vi "DP-Init Level Series.vi"(0 "state":T2, 1 "DP Freqs":T6, 5 "Parameters":T3, 11 "error in (no error)":errorcluster) -> (8 "level series":T1, 14 "Nominal f2 SPL":dbl[](array[numeric]), 15 "error out":errorcluster)   [LabVIEW 2020]
uses:
  Typedefs/DP-Freqs.ctl
  Typedefs/DP-Parameters.ctl
  Typedefs/DP-Stimulus Params.ctl
  Typedefs/DP-Response Params.ctl
  Typedefs/DP-Runtime State.ctl
  Typedefs/DP-Level Series Info.ctl
  epl-vi-lib/Utility VIs/Math VIs/LinSpace (start-stop-step).vi
  Calibration VIs/CIE-2 Tone.vi
panel:
  out "Nominal f1 SPL":dbl[](array[numeric])
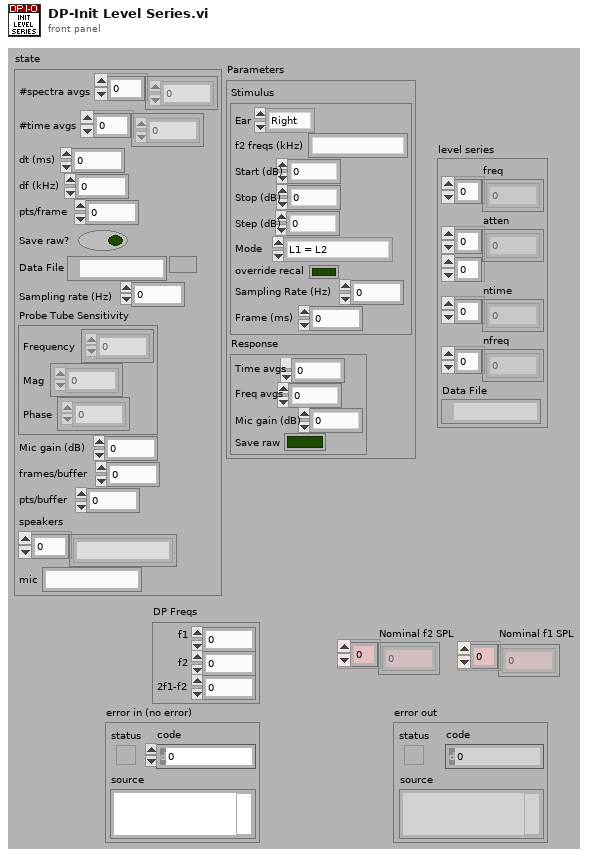
[diagram p1: front panel]
types:
  T1 = typedef "DP-Level Series Info.ctl" = cluster{"freq":dbl[], "atten":dbl[][], "ntime":i32[], "nfreq":i32[], "Data File":path}
  T2 = typedef "DP-Runtime State.ctl" = cluster{"#spectra avgs":i32[], "#time avgs":i32[], "dt (ms)":dbl, "df (kHz)":dbl, "pts/frame":i32, "Save raw?":bool, "Data File":path, "Sampling rate (Hz)":dbl, "Probe Tube Sensitivity":cluster{"Frequency":dbl[], "Mag":dbl[], "Phase":dbl[]}, "Mic gain (dB)":dbl, "frames/buffer":i32, "pts/buffer":i32, "speakers":string[], "mic":string}
  T3 = typedef "DP-Parameters.ctl" = cluster{"Stimulus":T4, "Response":T5}
  T4 = typedef "DP-Stimulus Params.ctl" = cluster{"Ear":enum16{"Right", "Left"}, "f2 freqs (kHz)":string, "Start (dB)":dbl, "Stop (dB)":dbl, "Step (dB)":dbl, "Mode":enum16{"L1 = L2", "L1 = L2 + 10 dB"}, "override recal":bool, "Sampling Rate (Hz)":dbl, "Frame (ms)":dbl}
  T5 = typedef "DP-Response Params.ctl" = cluster{"Time avgs":i32, "Freq avgs":i32, "Mic gain (dB)":dbl, "Save raw":bool}
  T6 = typedef "DP-Freqs.ctl" = cluster{"f1":dbl, "f2":dbl, "2f1-f2":dbl}
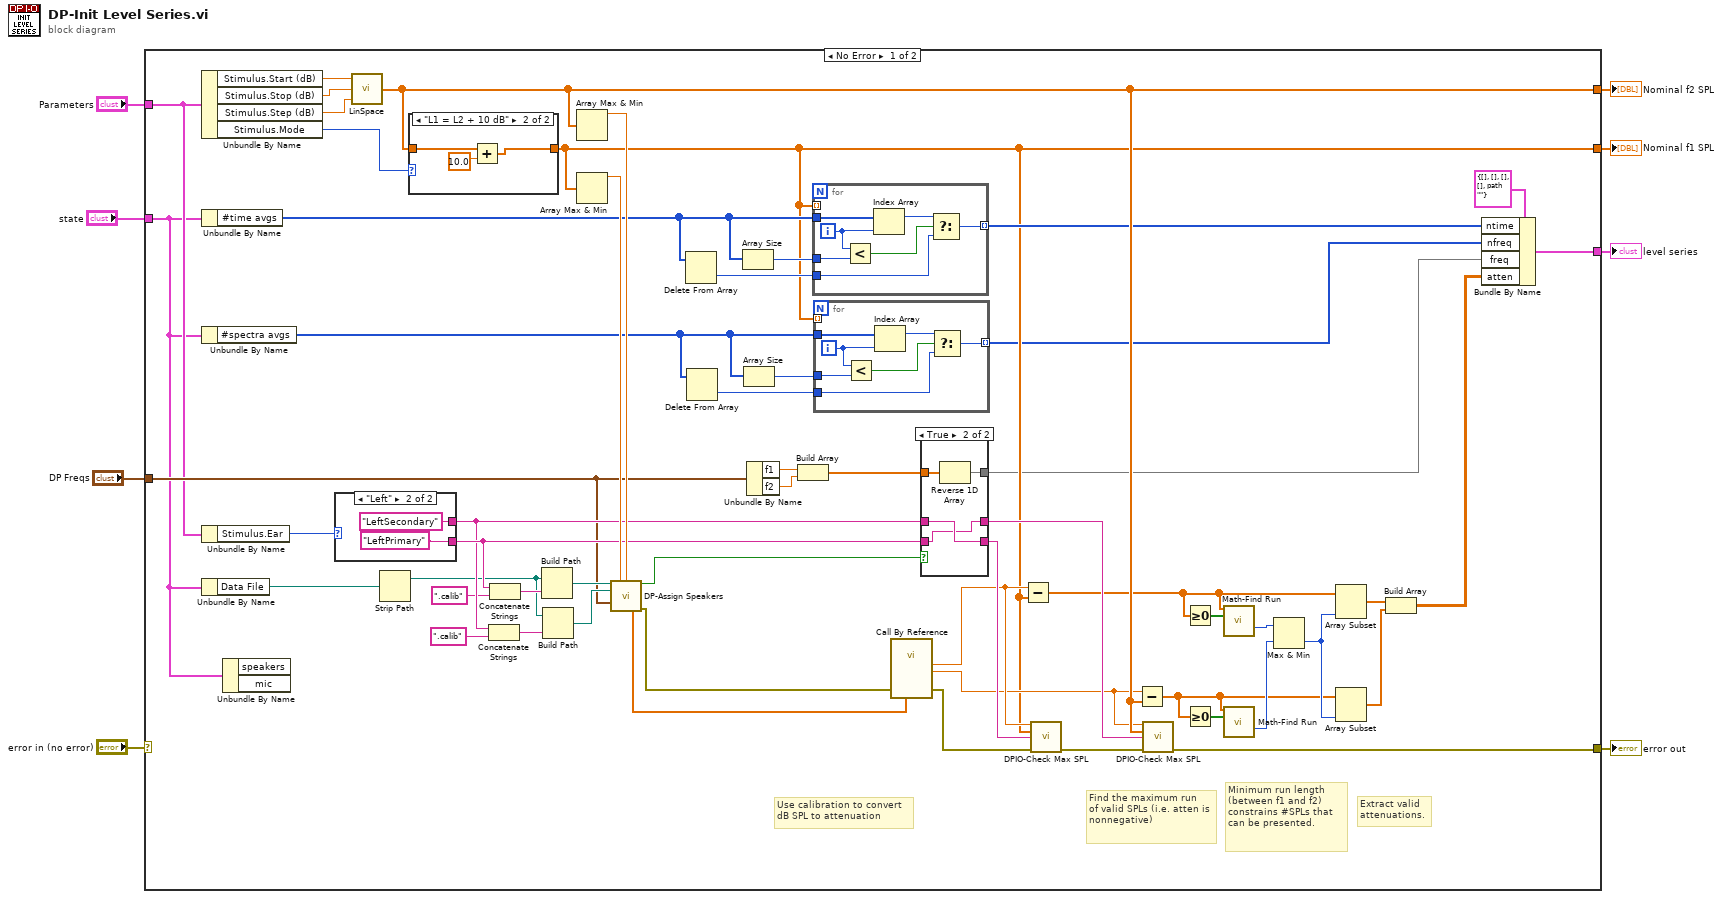
[diagram p0: block diagram]
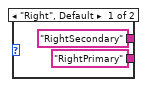
[diagram p3: hidden frame]
diagram:
  n1 = case shown="No Error" "error in (no error)" {
    selector: "error in (no error)" -> [_ w94]
    tunnel: "Parameters" -> [w24 _]
    tunnel: [w64 w94] -> w8
    tunnel: "DP Freqs" -> [w28 _]
    tunnel: "state" -> [w9 _]
    tunnel: [w43 _] -> w3
    tunnel: [w15 _] -> w2
    tunnel: [w10 _] -> w1
    frame No Error {
      # "Extract valid attenuations."
      # "Minimum run length (between f1 and f2) constrains #SPLs that can be presented."
      # "Find the maximum run\nof valid SPLs (i.e. atten is nonnegative)"
      # "Use calibration to convert\ndB SPL to attenuation"
      n2 = Unbundle By Name(w24) -> ("Stimulus.Start (dB)"=w63:dbl, "Stimulus.Stop (dB)"=w62:dbl, "Stimulus.Step (dB)"=w61:dbl, "Stimulus.Mode"=w60:enum16{"L1 = L2", "L1 = L2 + 10 dB"})
      n3 = Unbundle By Name(w9) -> ("#time avgs"=w18:i32[])
      n4 = Unbundle By Name(w9) -> ("#spectra avgs"=w14:i32[])
      n5 = Unbundle By Name(w24) -> ("Stimulus.Ear"=w23:enum16{"Right", "Left"})
      n6 = Unbundle By Name(w9) -> ("Data File"=w42:path)
      n7 = Unbundle By Name(w9) -> ()  [unwired: 2 out]
      n8 = case shown="\"Left\"" w23 {
        tunnel: ["RightPrimary" "LeftPrimary"] -> w54
        tunnel: ["RightSecondary" "LeftSecondary"] -> w52
        frame "Right", Default {
        }
        frame "Left" {
        }
      }
      n9 = call-poly "LinSpace.vi"("Step"=w61, "Stop"=w62, "Start"=w63) -> ("Array"=w43:dbl[])  [unwired: 1 in, 1 out]
      n10 = Strip Path(path=w42) -> (stripped path=w47:path)  [unwired: 1 out]
      n11 = case shown="\"L1 = L2 + 10 dB\"" w60 {
        tunnel: w43 -> [w90 w93]
        tunnel: [w90 w91] -> w15
        frame "L1 = L2", Default {
        }
        frame "L1 = L2 + 10 dB" {
          n12 = Add(x=w93, y=10.0 ("Numeric")) -> (x+y=w91:dbl[])
        }
      }
      n13 = Concatenate Strings(w52, ".calib" ("string")) -> (w53:string)
      n14 = Concatenate Strings(w54, ".calib" ("string")) -> (w55:string)
      n15 = Build Path(base path=w47, name or relative path=w55) -> (appended path=w49:path)
      n16 = Build Path(base path=w47, name or relative path=w53) -> (appended path=w48:path)
      n17 = Array Max & Min(array=w43) -> (max value=w58:dbl)  [unwired: 3 out]
      n18 = Array Max & Min(array=w15) -> (max value=w57:dbl)  [unwired: 3 out]
      n19 = call "DP-Assign Speakers.vi"("Primary"=w49, "F1 Max Req"=w57, "F2 Max  Req"=w58, "Secondary"=w48, "DP Freqs"=w28) -> ("Flipped?"=w44:bool, "Nominal Max SPL"=w56:dbl[], "error out"=w59:errorcluster)  [unwired: 8 in]
      n20 = Delete From Array(array=w18) -> (deleted portion=w22:i32)  [unwired: 2 in, 1 out]
      n21 = Delete From Array(array=w14) -> (deleted portion=w17:i32)  [unwired: 2 in, 1 out]
      n22 = Array Size(array=w18) -> (size(s)=w21:i32)
      n23 = Array Size(array=w14) -> (size(s)=w16:i32)
      n24 = Unbundle By Name(w28) -> ("f1"=w27:dbl, "f2"=w26:dbl)
      n25 = Build Array(w27, w26) -> (w25:dbl[])
      n26 = for {
        tunnel: w18 -> [w76]
        tunnel: w15 -> [_] mode=indexing
        tunnel: w22 -> [w75]
        tunnel: w21 -> [w78]
        tunnel: [w72] -> w19 mode=indexing
        i -> [w73]
        n27 = Less?(x=w73, y=w78) -> (x < y?=w77:bool)
        n28 = Index Array(array=w76, index=w73) -> (element=w74:i32)
        n29 = Select(t=w74, s=w77, f=w75) -> (s? t:f=w72:i32)
      }
      n30 = for {
        tunnel: w14 -> [w69]
        tunnel: w17 -> [w68]
        tunnel: w16 -> [w71]
        tunnel: [w65] -> w13 mode=indexing
        tunnel: w15 -> [_] mode=indexing
        i -> [w66]
        n31 = Less?(x=w66, y=w71) -> (x < y?=w70:bool)
        n32 = Index Array(array=w69, index=w66) -> (element=w67:i32)
        n33 = Select(t=w67, s=w70, f=w68) -> (s? t:f=w65:i32)
      }
      n34 = call-by-ref "?"("error in (no error)"=w59, "Nominal Max SPLs"=w56) -> ("Max SPL1"=w30:dbl, "Max SPL2"=w29:dbl, "error out"=w38:errorcluster)  [unwired: 13 in, 2 out]
      n35 = case shown="True" w44 {
        tunnel: w54 -> [w80 w84]
        tunnel: w52 -> [w81 w85]
        tunnel: [w81 w84] -> w46
        tunnel: [w80 w85] -> w45
        tunnel: w25 -> [w79 w83]
        tunnel: [w79 w82] -> w12
        frame False {
        }
        frame True {
          n36 = Reverse 1D Array(array=w83) -> (reversed array=w82:dbl[])
        }
      }
      n37 = Subtract(x=w30, y=w15) -> (x-y=w35:dbl[])
      n38 = call "DPIO-Check Max SPL.vi"("Max SPL"=w30, "SPL Array"=w15, "Channel"=w45, "error in (no error)"=w38) -> ("error out"=w31:errorcluster)  [unwired: 11 in]
      n39 = Subtract(x=w29, y=w43) -> (x-y=w34:dbl[])
      n40 = call "DPIO-Check Max SPL.vi"("Max SPL"=w29, "SPL Array"=w43, "Channel"=w46, "error in (no error)"=w31) -> ("error out"=w64:errorcluster)  [unwired: 11 in]
      n41 = Greater Or Equal To 0?(x=w35) -> (x >= 0?=w41:bool[])
      n42 = Greater Or Equal To 0?(x=w34) -> (x >= 0?=w32:bool[])
      n43 = call "Math-Find Run.vi"("Array"=w35, "Condition"=w41) -> ("Run length"=w40:i32)  [unwired: 10 in, 3 out]
      n44 = call "Math-Find Run.vi"("Array"=w34, "Condition"=w32) -> ("Run length"=w39:i32)  [unwired: 10 in, 3 out]
      n45 = Max & Min(x=w40, y=w39) -> (min(x,y)=w37:i32)  [unwired: 1 out]
      n46 = Array Subset(array=w35, length=w37) -> (w36:dbl[])  [unwired: 1 in]
      n47 = Array Subset(array=w34, length=w37) -> (w33:dbl[])  [unwired: 1 in]
      n48 = Build Array(w36, w33) -> (w11:dbl[][])
      n49 = Bundle By Name(cluster=T1 {"freq"=[], "atten"=[], "ntime"=[], "nfreq"=[], "Data File"=path ""} ("level series"), "ntime"=w19, "nfreq"=w13, "freq"=w12, "atten"=w11) -> (w10:T1)
    }
    frame Error {
    }
  }
  "error out" <- w8
  "Nominal f1 SPL" <- w2
  "Nominal f2 SPL" <- w3
  "level series" <- w1
